vi "Confirm Sub-Block.vi"(8 "error in":errorcluster, 11 "Block Upload Transfer in":refnum<class "Block Upload Sub-Block Transfer.lvclass">) -> (0 "error out":errorcluster, 3 "Block Upload Transfer out":refnum<class "Block Upload Sub-Block Transfer.lvclass">)   [LabVIEW 2020, in "CANopen.lvlib" / "SDO Manager.lvlib" / "Block Upload Sub-Block Transfer.lvclass"]
uses:
  Block Upload Sub-Block Transfer.lvclass
  Block Upload Sub-Block Transfer.lvclass/Block Upload Sub-Block Transfer.ctl
  HAL/Source/Interfaces/ICommunicate/ICommunicate.lvclass
  CANopen Message/CANopen Message.lvclass
  Typedefs/Function Code.ctl
  CANopen.lvlib
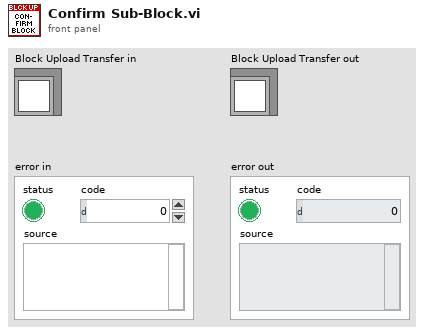
[diagram p1: front panel]
types:
  T1 = typedef "CANopen.lvlib/Function Code.ctl" = u8
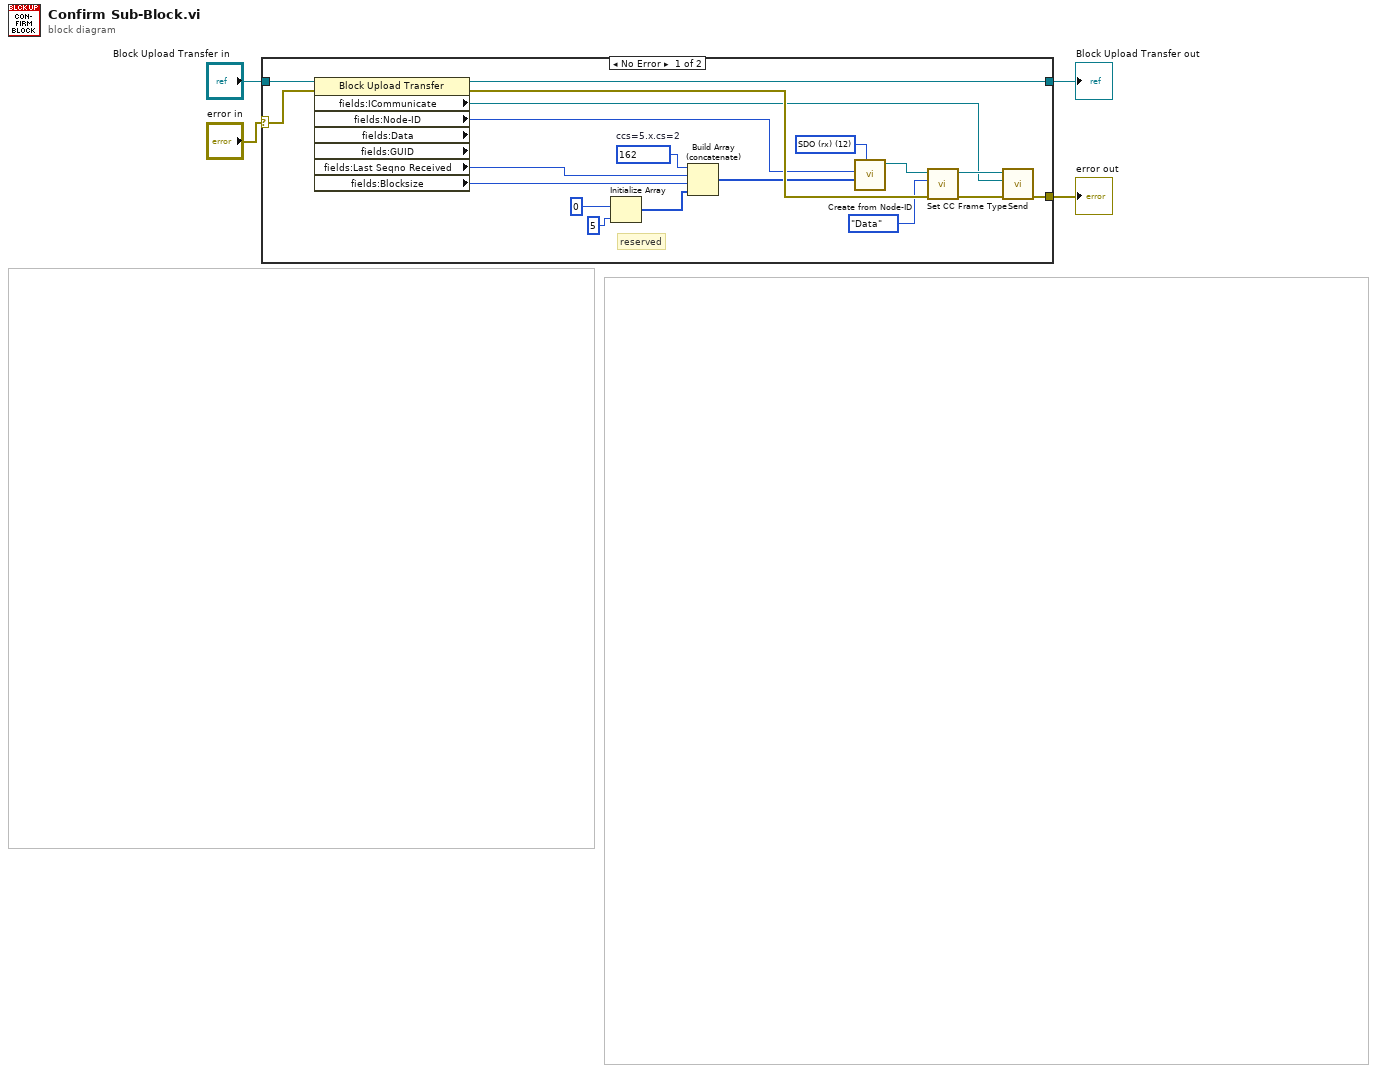
[diagram p0: block diagram]
diagram:
  n1 = case shown="No Error" "error in" {
    selector: "error in" -> [w22 w24]
    tunnel: "Block Upload Transfer in" -> [w21 w25]
    tunnel: [w20 w25] -> w1
    tunnel: [w19 w24] -> w2
    frame No Error {
      w14 = T1 12 items=["NMT"=0, "EMCY/SYNC"=1, "TIME"=2, "PDO1 (tx)"=3, "PDO1 (rx)"=4, "PDO2 (tx)"=5, "PDO2 (rx)"=6, "PDO3 (tx)"=7, "PDO3 (rx)"=8, "PDO4 (tx)"=9, "PDO4 (rx)"=10, "SDO (tx)"=11, "SDO (rx)"=12, "NMT error control"=14] ("Function Code")
      w17 = u8 162  # ccs=5.x.cs=2
      # "reserved"
      n2 = property class="Block Upload Transfer" props=["fields:ICommunicate", "fields:Node-ID", "fields:Data", "fields:GUID", "fields:Last Seqno Received", "fields:Blocksize"](reference=w21, error in=w22) -> (reference out=w20:refnum<class "Block Upload Sub-Block Transfer.lvclass">, error out=w23:errorcluster, "fields:ICommunicate"=w9:refnum<class "ICommunicate.lvclass">, "fields:Node-ID"=w18:u8, "fields:Last Seqno Received"=w8:u8, "fields:Blocksize"=w7:u8)  [unwired: 2 out]
      n3 = Initialize Array(u8 0, 5 ("y")) -> (w6:u8[])
      n4 = Build Array (concatenate)(w17, w8, w7, w6) -> (w15:u8[])
      n5 = call "Create from Node-ID.vi"("Function Code"=w14, "Data"=w15, "Node-ID"=w18) -> ("CANopen Message"=w13:refnum<class "CANopen Message.lvclass">)  [unwired: 8 in]
      n6 = call "Set CC Frame Type.vi"("error in"=w23, "CC Frame Type"=enum8{"Data", "Remote", "Error", "Overload"}."Data", "CANopen Message in"=w13) -> ("error out"=w12:errorcluster, "CANopen Message out"=w11:refnum<class "CANopen Message.lvclass">)  [unwired: 7 in]
      n7 = call "Send.vi"("error in"=w12, "ICommunicate"=w9, "CANopen Message in"=w11) -> ("error out"=w19:errorcluster)  [unwired: 7 in, 1 out]
    }
    frame Error {
    }
  }
  "Block Upload Transfer out" <- w1
  "error out" <- w2
